vi "01.Evd.1_Ask.3.vi"() -> ()   [LabVIEW 2025]
panel:
  in  "Tank Control":dbl(slide) scale=0.0..155.0
  out "Led 2":bool caption="Boolean 4"
  out "Meter":dbl(knob) scale=0.0..180.0
  out "Boolean 2":bool caption="Led 1"
  in  "Led Control 1":bool
  in  "Led Control 2":bool
  in  "Thermometer\nControl":dbl(slide) scale=0.0..14.0
  in  "stop":bool
  out "Tank":dbl(slide) scale=0.0..155.0
  out "Thermometer":dbl(slide) scale=0.0..14.0
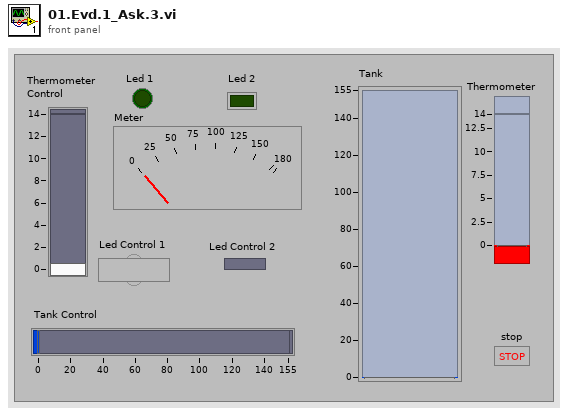
[diagram p1: front panel]
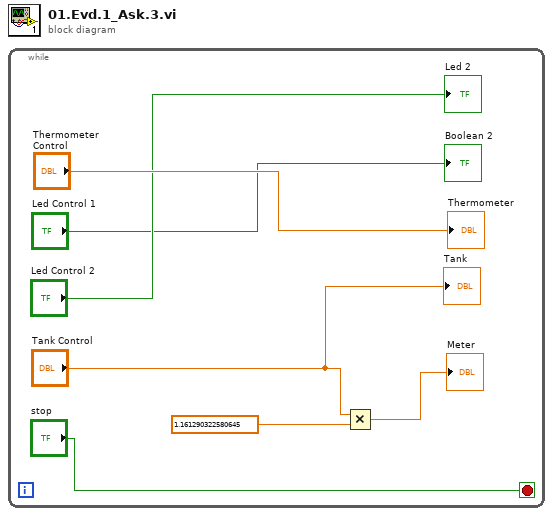
[diagram p0: block diagram]
diagram:
  n1 = while {
    stop <- "stop" stop-if-true
    n2 = Multiply(x="Tank Control", y=1.161290322580645) -> (x*y=→"Meter":dbl)
    "Thermometer" <- "Thermometer\nControl"
    "Tank" <- "Tank Control"
    "Boolean 2" <- "Led Control 1"
    "Led 2" <- "Led Control 2"
  }
